vi "waypoints_to_queue.vi"(10 "Waypoint queue":refnum<queue>, 11 "WP array":refnum<class "Waypoint.lvclass">[](array[class])) -> (3 "Waypoint queue OUT":refnum<queue>)   [LabVIEW 2013]
doc: "This VI takes a waypoint array and adds it to the waypoint queue, where the points are added to the front off the back of the array. Example:\n\nQueue = 1, 2, 3, 4\nArray = a, b, c, d\n\nAfterwards, queue will be = a, b, c, d, 1, 2, 3, 4\n\nEric Schneider, September 2014"
uses:
  Classes/Waypoint/Waypoint.lvclass
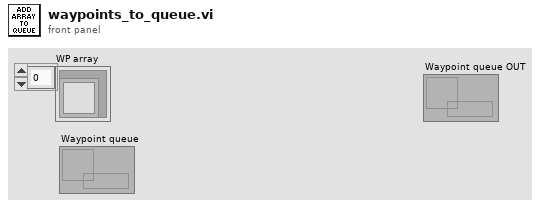
[diagram p1: front panel]
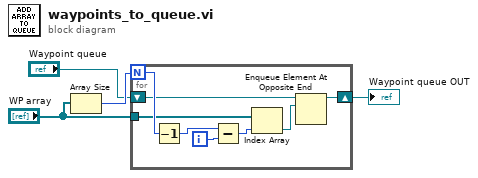
[diagram p0: block diagram]
diagram:
  n1 = Array Size(array="WP array") -> (size(s)=w4:i32)
  n2 = for {
    N: w4 -> [w12]
    tunnel: "WP array" -> [w8]
    shift-right: [w5] -> w1
    shift-left: "Waypoint queue" -> [w7]
    i -> [w10]
    n3 = Decrement(x=w12) -> (x-1=w11:i32)
    n4 = Subtract(x=w11, y=w10) -> (x-y=w9:i32)
    n5 = Index Array(array=w8, index=w9) -> (element=w6:refnum<class "Waypoint.lvclass">)
    n6 = Enqueue Element At Opposite End(queue=w7, element=w6) -> (queue out=w5:refnum<queue>)  [unwired: 2 in, 2 out]
  }
  "Waypoint queue OUT" <- w1
